vi "5_0_inverse FFT of one sided vs two sided spectrum.vi"() -> ()   [LabVIEW 2009]
uses:
  <vilib>/measure/matone.llb/Extract Single Tone Information 1 Chan.vi
  <vilib>/Analysis/2dsp.llb/Inverse Complex FFT.vi
  <vilib>/Analysis/2dsp.llb/Real FFT.vi
  <vilib>/Analysis/NI_AALBase.lvlib
  <vilib>/measure/NI_MAPro.lvlib
  <vilib>/Analysis/NI_AALPro.lvlib
panel:
  out "PHASE PLOT OF IFFT":dbl[](graph)=[-0.8524697408335709, -0.40748488207664046, -0.1268654978335297, 0.12686549783352957, 0.40748488207664024, 0.8524697408335707, 1.5889194659707906, 1.5966731628316637, 1.6041910783639635, 1.6118107017257388, 1.6197123575445933, 1.6280401156686646, 1.6369385301034163, 1.6465715078080854, 1.6571380811494125, 1.668890797356469, 1.6821610796097555, 1.6973972432967555, 1.715224596602943, 1.7365449259694004, 1.7627092545662675, 1.7958345210056603, 1.8394218293357656, 1.8996554825655303, 1.9883658653105416, 2.130300389496201, 2.380319581783001, 2.8348234385781517, 3.4483618686014315, 3.9028657253965804, 4.152884917683385, 4.294819441869041, 4.383529824614057, 4.443763477843824, 4.487350786173925, 4.520476052613318, 4.546640381210186, 4.567960710576643, 4.58578806388283, 4.60102422756983, 4.614294509823115, 4.626047226030174, 4.636613799371501, 4.64624677707617, 4.655145191510922, 4.6634729496349925, 4.671374605453847, 4.678994228815623, 4.6865121443479225, 4.694265841208795]
  out "PHASE PLOT OF IFFT":dbl[](graph)=[7.806255641895632e-18, -1.070222432237112e-16, -6.926012986585332e-17, -8.95286082736778e-17, -2.4757524506244172e-17, -7.708860338443508e-17, -1.1870100966642376e-16, -2.028583387333138e-17, -3.244626402670354e-17, -5.1237142864996e-17, -2.7729818653163923e-17, -3.052166662838311, -3.857180626159561, -3.4522573371371315, -2.9265484443936347, -3.332323038985992, -3.763563654552602, -6.34621297924532, -3.609239564041977, -1.9564428913976795, -1.3853313030041945, -3.745235757916132, -4.725507827503854, -5.486763286525393, -6.081674965765823, -6.218075312241696, -8.383184554491082, -6.174127459644382, -4.966447680000442, -6.573210745577857, -6.291926051943064, -6.7495541302012425, -6.759313157449682, -7.183594302336601, -6.596101120448532, -4.71238898038469, -6.242738848645043, -3.7248642537017105, -6.79886173291, -9.657554622227867, -7.853981633974483, -9.366981075199789, -9.552737084476966, -9.533582055953655, -9.277382354528344, -9.699789856635407, -7.853981633974483, -5.43623840730894, -7.060585609857342, -7.853981633974483, -6.7066247133393055, -6.738371234650006, -6.341312119269376, -6.200689197407941, -6.556801127375861, -7.853981633974483, -6.550303780412898, -6.35585762397127, -4.71238898038469, -3.6541253373308886, -4.71238898038469, -3.8318672767363133, -5.119942186117699, -3.710928254072696, -4.119135738411837, -3.7280195380119254, -4.2843202387005626, -1.9811033120489254, 0.689526342512747, -0.5330510016729039, 2.3244728172082056, 0.12183125310633174, -2.5660264286125947, -0.6175294809935509, -2.542876117116644, 0.0480981026284778, -1.3910453138610972, -3.2703822235332276, -2.884076452454559, -2.9596871114658927, -3.1595659301998222, -3.734802108132001, -3.5839862787232537, -3.8616075510042385, -3.6946513573707214, -4.71238898038469, -4.132634099636267, -6.053086329873605, -3.050702272396979, -3.737803844028845, -4.71238898038469, -5.601427829621794, -7.853981633974483, -6.530132536286139, -6.270083843304302, -6.450892009584458, -4.71238898038469, -2.7386471933636867, -2.0312901374214394, -3.9961826176864443]
  out "MAGNITUDE OF IFFT":dbl[](graph)=[0.01, 0.01, 0.01, 0.01, 0.01, 0.01, 0.01, 0.009999999999999998, 0.01, 0.01, 0.01, 1.1769286549004275e-18, 6.6460045320375995e-19, 1.3282359395858361e-18, 6.149476416360019e-19, 8.252020219132452e-19, 6.110656010294029e-19, 4.828187813833805e-19, 1.7839634152204216e-19, 1.266411875170956e-19, 3.615896476700937e-19, 3.9137843402403226e-19, 5.475363318400623e-19, 6.697102589357712e-19, 8.766988196791402e-19, 8.153536263231808e-19, 2.8656933719989682e-19, 6.348449873238717e-19, 5.516249800940764e-19, 4.568959162104949e-19, 1.0766538855279154e-18, 6.214814302944858e-19, 9.36869293875907e-19, 8.934827920481643e-19, 5.834435124906911e-19, 3.345487400322162e-20, 5.555658799234696e-19, 3.3253541146592564e-19, 3.1904450819839834e-19, 5.70498058306926e-19, 3.129593843111334e-19, 1.3900999350287225e-19, 2.798436470622704e-19, 9.77223791795179e-19, 9.820940712407218e-19, 4.3258949649040544e-19, 2.3589867581032264e-19, 2.0954758884453495e-19, 1.947105335811547e-19, 3.18890963982299e-19, 1.8998013584594692e-19, 1.2360817255724467e-18, 1.11210123854733e-18, 1.1140116385727674e-18, 1.1531188793745111e-18, 3.276667140500816e-19, 1.1510442472719137e-18, 1.1131611811269628e-18, 4.0650087380757416e-20, 1.2739142380935128e-18, 2.7729818653163923e-19, 1.2385093013585569e-18, 2.6191158553915634e-19, 6.569021055880242e-19, 6.516135414902478e-19, 7.161697525459617e-19, 7.517127896064829e-19, 2.8046798059658494e-19, 6.469331065721965e-19, 6.205367602260962e-19, 4.87382582781785e-19, 4.775392787866618e-19, 2.8336606694979876e-19, 1.440340997375154e-19, 8.810147345899317e-20, 3.0833776940221066e-19, 1.747274344599814e-19, 1.0334689731741024e-18, 1.6467217117304525e-19, 3.1673065223925814e-19, 5.236186963063961e-19, 6.6949404246627545e-19, 9.2136777446432e-19, 7.38380600284519e-19, 6.523649036422596e-19, 4.444643355793925e-19, 1.0133121096240545e-18, 1.4253454335586116e-18, 1.3935308412180152e-18, 6.708547467780006e-19, 3.129593843111334e-19, 8.936502141247432e-19, 3.1326666521253046e-19, 1.0018377239596355e-18, 4.16369368281998e-19, 7.037630734670443e-19, 2.3589867581032264e-19, 7.5430140173610385e-19, 3.122881064119443e-19, 4.227631070529326e-19]
  out "MAGNITUDE OF IFFT":dbl[](graph)=[0.030085439591800364, 0.021565797340465785, 0.01996041465777327, 0.019960414657773266, 0.02156579734046578, 0.030085439591800368, 0.011036219870674057, 0.007729782799349668, 0.005990078353216028, 0.004877706510838509, 0.00409027017264813, 0.0034957376876723805, 0.003025993855965793, 0.002641914167007991, 0.0023192569390351535, 0.0020421243943848154, 0.0017996178995784938, 0.0015839953294540714, 0.0013895964663497536, 0.0012121894116278009, 0.0010485639705040803, 0.0008962838542587668, 0.0007535610909382819, 0.000619264966236809, 0.0004931695725765839, 0.0003768139253352483, 0.0002762589760916794, 0.00020979442545002608, 0.00020979442545002614, 0.0002762589760916788, 0.0003768139253352492, 0.0004931695725765836, 0.00061926496623681, 0.0007535610909382812, 0.0008962838542587682, 0.0010485639705040805, 0.0012121894116277985, 0.001389596466349754, 0.0015839953294540714, 0.001799617899578496, 0.0020421243943848167, 0.002319256939035153, 0.0026419141670079908, 0.003025993855965793, 0.0034957376876723774, 0.004090270172648129, 0.0048777065108385085, 0.005990078353216027, 0.007729782799349666, 0.011036219870674059]
  out "IMAGINARY PART OF IFFT":dbl[](graph)=[-0.022651571147094166, -0.008546555734916897, -0.0025255006058700186, 0.002525500605870015, 0.008546555734916892, 0.022651571147094166, 0.011034407507150573, 0.0077271949713412814, 0.005986738567673323, 0.004873604498302707, 0.004085377593963007, 0.003490011745111045, 0.0030193772232602416, 0.002634333021058182, 0.0023106173956894526, 0.0020323070737813097, 0.001788469900357093, 0.0015713183012147198, 0.0013751284810124915, 0.001195576500966188, 0.0010293135577846436, 0.0008736845811875991, 0.0007265358337866712, 0.0005860794301187135, 0.00045079510569145584, 0.0003193567508704931, 0.00019057550176038718, 6.335377612981474e-05, -6.335377612981419e-05, -0.00019057550176038586, -0.00031935675087049384, -0.000450795105691455, -0.0005860794301187146, -0.0007265358337866712, -0.0008736845811876004, -0.0010293135577846436, -0.0011955765009661857, -0.001375128481012492, -0.0015713183012147196, -0.001788469900357095, -0.0020323070737813106, -0.002310617395689452, -0.0026343330210581817, -0.0030193772232602416, -0.0034900117451110418, -0.004085377593963006, -0.0048736044983027065, -0.0059867385676733225, -0.007727194971341279, -0.011034407507150573]
  out "IMAGINARY  PART OF IFFT":dbl[](graph)=[7.806255641895632e-20, -1.070222432237112e-18, -6.926012986585332e-19, -8.95286082736778e-19, -2.475752450624417e-19, -7.708860338443508e-19, -1.1870100966642376e-18, -2.0285833873331376e-19, -3.2446264026703544e-19, -5.1237142864996e-19, -2.7729818653163923e-19, -1.051077888933472e-19, 4.3601862232782005e-19, 4.0603052899077807e-19, -1.312240581677739e-19, 1.564385695482534e-19, 3.5603015337493493e-19, -3.0410800064616527e-20, 8.04187682809416e-20, -1.1734007814767696e-19, -3.5538860391659286e-19, 2.2216420822923857e-19, 5.474892158783854e-19, 4.787482065753655e-19, 1.7547068906596255e-19, 5.3050169237540845e-20, -2.4736944495925564e-19, 6.909766737395167e-20, 5.339179868407177e-19, -1.3066154122079454e-19, -9.410636981189501e-21, -2.7944655499562363e-19, -4.294057449873437e-19, -7.001162107709157e-19, -1.7960384507442347e-19, 3.345487400322162e-20, 2.2464546137888218e-20, 1.8314639527799346e-19, -1.5732832051499322e-19, 1.316025965929817e-19, -3.129593843111334e-19, -8.029872339970768e-21, 3.5710909056241305e-20, 1.0611628763201875e-19, -1.4423277025846226e-19, 1.1747330538880442e-19, -2.3589867581032264e-19, 1.5700602710305712e-19, -1.365755924152834e-19, -3.18890963982299e-19, -7.806255641895632e-20, -5.434177655232912e-19, -6.460650408956147e-20, 9.179742081208677e-20, -3.115894503382571e-19, -3.276667140500816e-19, -3.038218141772169e-19, -8.082481524967397e-20, 4.0650087380757416e-20, 6.247097899101185e-19, 2.7729818653163923e-19, 7.886195098672507e-19, 2.404592958546189e-19, 3.5411790700049025e-19, 5.402699299637449e-19, 3.9632005538727372e-19, 6.838850975765389e-19, -2.5718869294115346e-19, 4.115606017225533e-19, -3.1533407612639655e-19, 3.5538860391659286e-19, 5.803539126420531e-20, -1.542389485149524e-19, -8.339901148187951e-20, -4.9652468088997603e-20, 1.482474413875035e-20, -1.7191226768039992e-19, 1.3273238009293602e-19, -4.1938616837222844e-20, -5.729784281695019e-20, 9.410636981189501e-21, 3.742639199761009e-19, 3.944411183458555e-19, 4.868851196889971e-19, 3.4268232578033095e-19, 4.444643355793925e-19, 8.477338263917479e-19, 3.250840823220212e-19, -1.264842323712848e-19, 3.766925804586781e-19, 3.129593843111334e-19, 5.631413846525491e-19, -3.1326666521253046e-19, -2.448941657101633e-19, 5.4548921803176945e-21, -1.1747330538880442e-19, 2.3589867581032264e-19, -2.9578390518120167e-19, -2.7975804181915034e-19, 3.18890963982299e-19]
  out "REAL PART OF IFFT":dbl[](graph)=[0.0198, 0.019800000000000005, 0.019800000000000005, 0.0198, 0.019800000000000005, 0.019800000000000005, -0.0001999999999999994, -0.0002000000000000014, -0.00019999999999999952, -0.00019999999999999977, -0.00020000000000000063, -0.00020000000000000196, -0.00020000000000000142, -0.000200000000000001, -0.0002000000000000014, -0.00019999999999999844, -0.00019999999999999952, -0.00019999999999999855, -0.00019999999999999955, -0.00020000000000000123, -0.00020000000000000234, -0.00019999999999999952, -0.00020000000000000004, -0.00020000000000000047, -0.00019999999999999898, -0.00019999999999999968, -0.00019999999999999944, -0.00019999999999999966, -0.0001999999999999999, -0.00019999999999999985, -0.00020000000000000025, -0.00020000000000000017, -0.00020000000000000017, -0.00019999999999999795, -0.00020000000000000017, -0.0002000000000000035, -0.00020000000000000052, -0.0001999999999999996, -0.0002000000000000001, -0.0001999999999999999, -0.00020000000000000196, -0.00020000000000000074, -0.00020000000000000074, -0.00020000000000000074, -0.00020000000000000074, -0.00020000000000000185, -0.000200000000000002, -0.00020000000000000172, -0.00020000000000000177, -0.00020000000000000302]
  out "REAL PART OF IFFT":dbl[](graph)=[0.01, 0.01, 0.01, 0.01, 0.01, 0.01, 0.01, 0.009999999999999998, 0.01, 0.01, 0.01, -1.1722258363641714e-18, -5.015790300461065e-19, -1.2646540715685605e-18, -6.007835288285301e-19, -8.102378360255736e-19, -4.966323576341414e-19, 4.818601030340264e-19, -1.5924219408380846e-19, -4.763713295358185e-20, 6.667843360785852e-20, -3.222113331355359e-19, 7.182839392716467e-21, 4.683075758779576e-19, 8.589591711516409e-19, 8.136259678145908e-19, -1.446732273910345e-19, 6.310734270223439e-19, 1.3864235280658389e-19, 4.378143897768028e-19, 1.0766127572781059e-18, 5.551115123125783e-19, 8.326672684688674e-19, 5.551115123125783e-19, 5.551115123125783e-19, 0.0, 5.551115123125783e-19, -2.7755575615628914e-19, 2.7755575615628914e-19, -5.551115123125783e-19, 0.0, -1.3877787807814457e-19, -2.7755575615628914e-19, -9.71445146547012e-19, -9.71445146547012e-19, -4.163336342344337e-19, 0.0, 1.3877787807814457e-19, 1.3877787807814457e-19, 0.0, 1.7320129705455935e-19, 1.1102230246251566e-18, 1.1102230246251566e-18, 1.1102230246251566e-18, 1.1102230246251566e-18, 0.0, 1.1102230246251566e-18, 1.1102230246251566e-18, 0.0, -1.1102230246251566e-18, 0.0, -9.549788260523884e-19, 1.0381235801548705e-19, -5.53281921146509e-19, -3.642919299551295e-19, -5.965144827743685e-19, -3.1204693776848427e-19, -1.11876111673348e-19, 4.991395751580141e-19, 5.344439083995734e-19, -3.335276933108533e-19, 4.739996372835065e-19, -2.3771132631744684e-19, 1.174326478073362e-19, -7.277707082808949e-20, 3.079811796216636e-19, 3.12385750947386e-20, -1.0249098661777034e-18, -1.5924219408380846e-19, -3.115048366822415e-19, -5.23534124038938e-19, -5.551115123125783e-19, -8.326672684688674e-19, -5.551115123125783e-19, -5.551115123125783e-19, 0.0, -5.551115123125783e-19, 1.3877787807814458e-18, -1.3877787807814458e-18, -5.551115123125783e-19, 0.0, 6.938893903907229e-19, 0.0, 9.71445146547012e-19, 4.163336342344337e-19, 6.938893903907229e-19, 0.0, -6.938893903907229e-19, -1.3877787807814457e-19, -2.7755575615628914e-19]
  out "FREQ":dbl=0.049366588097272006 format="%.2p"
  out "FREQ":dbl=0.02469635114895025 format="%.2p"
  out "?":bool
  out "?":bool
  out "INVERSE FFT OF ONE SIDED SPECTRUM":cluster{i32, dbl, dbl[]}(graph)={0, 0.001, [0.0198, 0.019800000000000005, 0.019800000000000005, 0.0198, 0.019800000000000005, 0.019800000000000005, -0.0001999999999999994, -0.0002000000000000014, -0.00019999999999999952, -0.00019999999999999977, -0.00020000000000000063, -0.00020000000000000196, -0.00020000000000000142, -0.000200000000000001, -0.0002000000000000014, -0.00019999999999999844, -0.00019999999999999952, -0.00019999999999999855, -0.00019999999999999955, -0.00020000000000000123, -0.00020000000000000234, -0.00019999999999999952, -0.00020000000000000004, -0.00020000000000000047, -0.00019999999999999898, -0.00019999999999999968, -0.00019999999999999944, -0.00019999999999999966, -0.0001999999999999999, -0.00019999999999999985, -0.00020000000000000025, -0.00020000000000000017, -0.00020000000000000017, -0.00019999999999999795, -0.00020000000000000017, -0.0002000000000000035, -0.00020000000000000052, -0.0001999999999999996, -0.0002000000000000001, -0.0001999999999999999, -0.00020000000000000196, -0.00020000000000000074, -0.00020000000000000074, -0.00020000000000000074, -0.00020000000000000074, -0.00020000000000000185, -0.000200000000000002, -0.00020000000000000172, -0.00020000000000000177, -0.00020000000000000302]}
  out "INVERSE FFT OF TWO SIDED SPECTRUM":cluster{"index":i32, dbl, dbl[]}(graph)={"index"=0, 0.001, [0.01, 0.01, 0.01, 0.01, 0.01, 0.01, 0.01, 0.009999999999999998, 0.01, 0.01, 0.01, -1.1722258363641714e-18, -5.015790300461065e-19, -1.2646540715685605e-18, -6.007835288285301e-19, -8.102378360255736e-19, -4.966323576341414e-19, 4.818601030340264e-19, -1.5924219408380846e-19, -4.763713295358185e-20, 6.667843360785852e-20, -3.222113331355359e-19, 7.182839392716467e-21, 4.683075758779576e-19, 8.589591711516409e-19, 8.136259678145908e-19, -1.446732273910345e-19, 6.310734270223439e-19, 1.3864235280658389e-19, 4.378143897768028e-19, 1.0766127572781059e-18, 5.551115123125783e-19, 8.326672684688674e-19, 5.551115123125783e-19, 5.551115123125783e-19, 0.0, 5.551115123125783e-19, -2.7755575615628914e-19, 2.7755575615628914e-19, -5.551115123125783e-19, 0.0, -1.3877787807814457e-19, -2.7755575615628914e-19, -9.71445146547012e-19, -9.71445146547012e-19, -4.163336342344337e-19, 0.0, 1.3877787807814457e-19, 1.3877787807814457e-19, 0.0, 1.7320129705455935e-19, 1.1102230246251566e-18, 1.1102230246251566e-18, 1.1102230246251566e-18, 1.1102230246251566e-18, 0.0, 1.1102230246251566e-18, 1.1102230246251566e-18, 0.0, -1.1102230246251566e-18, 0.0, -9.549788260523884e-19, 1.0381235801548705e-19, -5.53281921146509e-19, -3.642919299551295e-19, -5.965144827743685e-19, -3.1204693776848427e-19, -1.11876111673348e-19, 4.991395751580141e-19, 5.344439083995734e-19, -3.335276933108533e-19, 4.739996372835065e-19, -2.3771132631744684e-19, 1.174326478073362e-19, -7.277707082808949e-20, 3.079811796216636e-19, 3.12385750947386e-20, -1.0249098661777034e-18, -1.5924219408380846e-19, -3.115048366822415e-19, -5.23534124038938e-19, -5.551115123125783e-19, -8.326672684688674e-19, -5.551115123125783e-19, -5.551115123125783e-19, 0.0, -5.551115123125783e-19, 1.3877787807814458e-18, -1.3877787807814458e-18, -5.551115123125783e-19, 0.0, 6.938893903907229e-19, 0.0, 9.71445146547012e-19, 4.163336342344337e-19, 6.938893903907229e-19, 0.0, -6.938893903907229e-19, -1.3877787807814457e-19, -2.7755575615628914e-19]}
  out "?":string="SAMPLE"
  in  "stop":bool
  out "DETECTED FREQUENCY":dbl=0.024696351148950267 format="%.2p"
  out "ONE SIDED FFT MAG PLOT":cluster{i32, dbl, dbl[]}(graph)={0, 10.0, [0.11, 0.2156827343158089, 0.20303192091000685, 0.1829258216733136, 0.156748090317914, 0.12627503029350087, 0.09353191720116408, 0.06063097450005466, 0.029605108344486146, 0.002251739098357606, 0.02, 0.03618768475694426, 0.045871861539495615, 0.04914626439933461, 0.04660229940576391, 0.03925221011010302, 0.028418967730971842, 0.015603755543126093, 0.0023436871809210187, 0.009927036344868552, 0.02, 0.026988776498658107, 0.03039054622059342, 0.03010869808349327, 0.026435786365307575, 0.02, 0.011681690419824685, 0.002509183429725328, 0.006455174897940613, 0.014227167303847467, 0.02, 0.023221284976236406, 0.023640737165832135, 0.02132473138039944, 0.016637294774129143, 0.01019050898988858, 0.002770324632154191, 0.004753846731831293, 0.011525926996682445, 0.016796071052742112, 0.02, 0.02081668504695303, 0.019198691928627776, 0.015372439512982547, 0.00980881455489394, 0.003167688806490725, 0.003777412316085198, 0.01022621260854057, 0.015440733616207286, 0.01882690532036019]}
  out "# OF CYCLES":dbl=5.0
  in  "?":bool
  out "TWO SIDED FFT MAG PLOT":cluster{"index":i32, dbl, dbl[]}(graph)={"index"=0, 10.0, [0.11, 0.10784136715790445, 0.10151596045500343, 0.0914629108366568, 0.078374045158957, 0.06313751514675044, 0.04676595860058204, 0.03031548725002733, 0.014802554172243073, 0.001125869549178803, 0.01, 0.01809384237847213, 0.022935930769747807, 0.024573132199667305, 0.023301149702881954, 0.01962610505505151, 0.014209483865485921, 0.0078018777715630466, 0.0011718435904605094, 0.004963518172434276, 0.01, 0.013494388249329053, 0.01519527311029671, 0.015054349041746636, 0.013217893182653788, 0.01, 0.005840845209912343, 0.001254591714862664, 0.0032275874489703063, 0.0071135836519237335, 0.01, 0.011610642488118203, 0.011820368582916067, 0.01066236569019972, 0.008318647387064572, 0.00509525449494429, 0.0013851623160770956, 0.0023769233659156467, 0.005762963498341223, 0.008398035526371056, 0.01, 0.010408342523476515, 0.009599345964313888, 0.0076862197564912735, 0.00490440727744697, 0.0015838444032453625, 0.001888706158042599, 0.005113106304270285, 0.007720366808103643, 0.009413452660180096, 0.01, 0.009413452660180096, 0.007720366808103643, 0.005113106304270285, 0.001888706158042599, 0.0015838444032453625, 0.00490440727744697, 0.0076862197564912735, 0.009599345964313888, 0.010408342523476515, 0.01, 0.008398035526371056, 0.005762963498341223, 0.0023769233659156467, 0.0013851623160770956, 0.00509525449494429, 0.008318647387064572, 0.01066236569019972, 0.011820368582916067, 0.011610642488118203, 0.01, 0.0071135836519237335, 0.0032275874489703063, 0.001254591714862664, 0.005840845209912343, 0.01, 0.013217893182653788, 0.015054349041746636, 0.01519527311029671, 0.013494388249329053, 0.01, 0.004963518172434276, 0.0011718435904605094, 0.0078018777715630466, 0.014209483865485921, 0.01962610505505151, 0.023301149702881954, 0.024573132199667305, 0.022935930769747807, 0.01809384237847213, 0.01, 0.001125869549178803, 0.014802554172243073, 0.03031548725002733, 0.04676595860058204, 0.06313751514675044, 0.078374045158957, 0.0914629108366568, 0.10151596045500343, 0.10784136715790445]}
  in  "Delta t":dbl=0.1 format="%0.2f"
  in  "Duty cycle (%)":dbl=50.0 format="%0.2f"
  in  "Width":i32=11
  in  "Start":dbl format="%0.2f"
  in  "End":dbl=1.0 format="%0.2f"
  out "TIME DOMAIN ORIGINAL SIGNAL":T1(graph)={0, "# OF SAMPLES"=1.0, "Sinc Pattern"=[1.0, 1.0, 1.0, 1.0, 1.0, 1.0, 1.0, 1.0, 1.0, 1.0, 1.0, 0.0, 0.0, 0.0, 0.0, 0.0, 0.0, 0.0, 0.0, 0.0, 0.0, 0.0, 0.0, 0.0, 0.0, 0.0, 0.0, 0.0, 0.0, 0.0, 0.0, 0.0, 0.0, 0.0, 0.0, 0.0, 0.0, 0.0, 0.0, 0.0, 0.0, 0.0, 0.0, 0.0, 0.0, 0.0, 0.0, 0.0, 0.0, 0.0, 0.0, 0.0, 0.0, 0.0, 0.0, 0.0, 0.0, 0.0, 0.0, 0.0, 0.0, 0.0, 0.0, 0.0, 0.0, 0.0, 0.0, 0.0, 0.0, 0.0, 0.0, 0.0, 0.0, 0.0, 0.0, 0.0, 0.0, 0.0, 0.0, 0.0, 0.0, 0.0, 0.0, 0.0, 0.0, 0.0, 0.0, 0.0, 0.0, 0.0, 0.0, 0.0, 0.0, 0.0, 0.0, 0.0, 0.0, 0.0, 0.0, 0.0]}
  in  "Reset phase":bool=TRUE
  in  "DELAY":dbl(knob) min=0.0 max=10.0 scale=0.0..10.0
  in  "SAMPLING\nFREQUENCY (Hz)":dbl(slide)=1000.0 scale=0.0..20000.0 scale format="%#_6p"
  in  "# OF SAMPLES":dbl=100.0
  in  "AMPLITUDE":dbl=1.0
  in  "PHASE IN":dbl(knob) scale=0.0..180.0
  in  "SIGNAL FREQUENCY":dbl(knob)=50.0 scale=0.0..10000.0 scale format="%#_6p"
  in  "SIGNAL":T2(ring)=enum."PULSE"
  # "SAMPLING INFO"
  # "ORIGINAL SIGNAL \nCHARACTERISTICS"
  # "RAMP"
  # "PULSE"
  # "SQUARE"
  # "SINC"
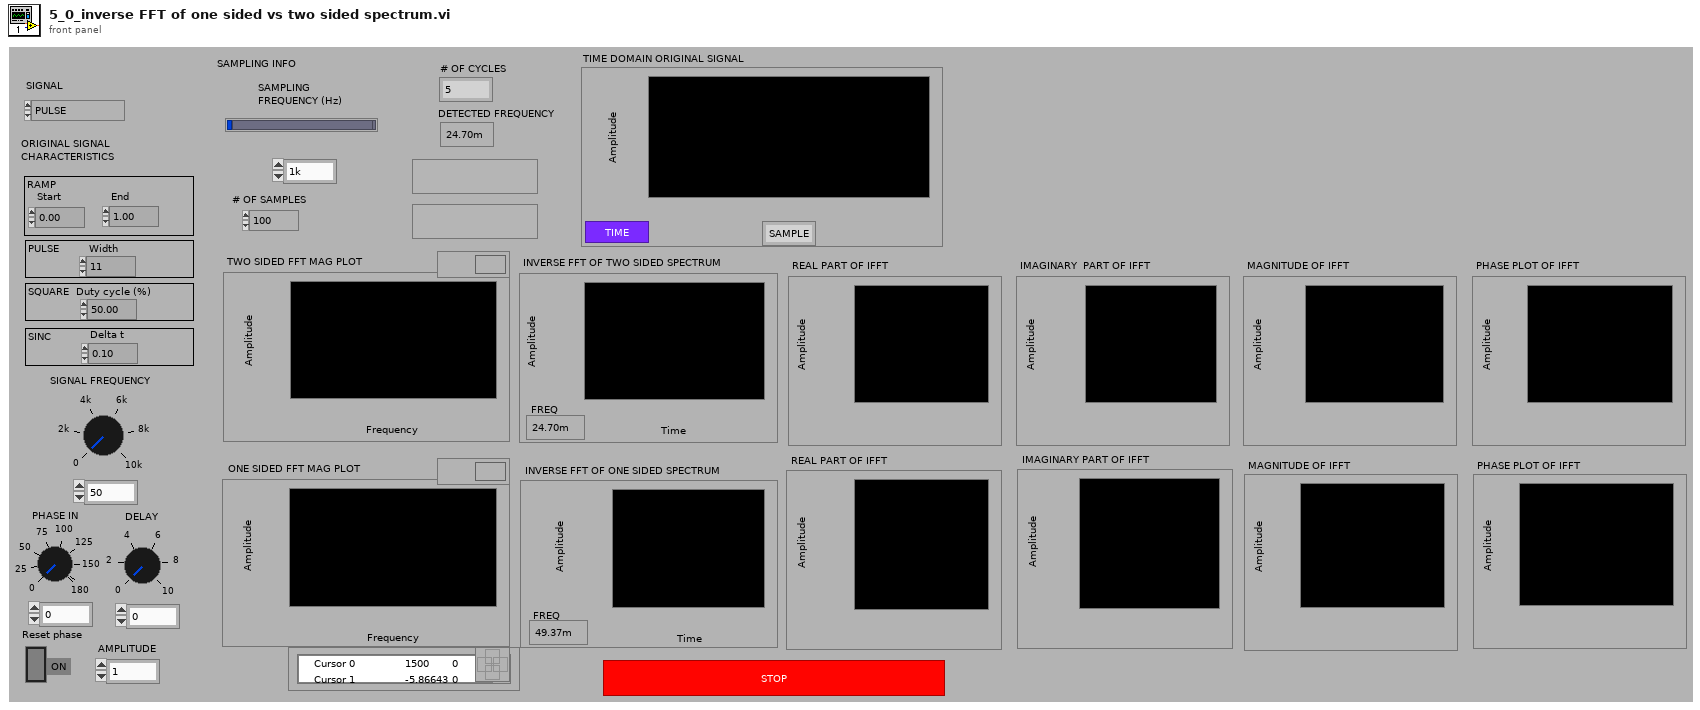
[diagram p1: front panel]
types:
  T1 = cluster{i32, "# OF SAMPLES":dbl, "Sinc Pattern":dbl[]}
  T2 = enum16{"SINE", "TRIANGULAR", "RAMP", "IMPULSE", "SINC ", "PULSE", "SQUARE"}
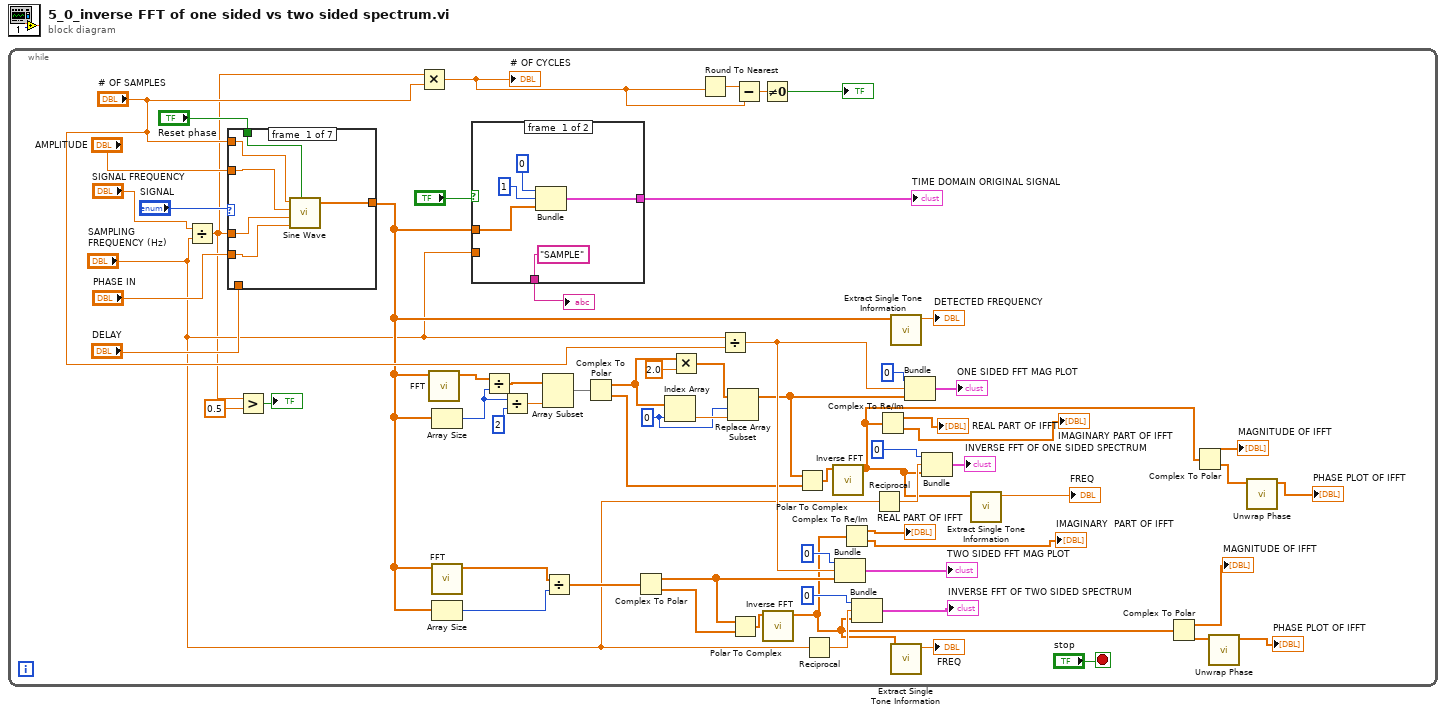
[diagram p0: block diagram]
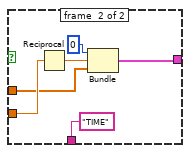
[diagram p2: hidden frame]
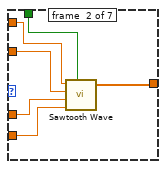
[diagram p3: hidden frame]
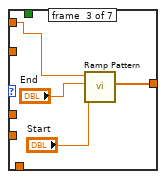
[diagram p4: hidden frame]
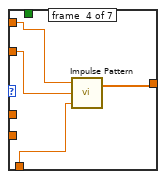
[diagram p5: hidden frame]
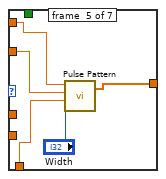
[diagram p6: hidden frame]
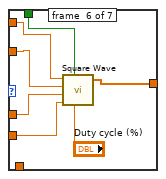
[diagram p7: hidden frame]
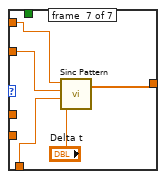
[diagram p8: hidden frame]
diagram:
  n1 = while {
    stop <- "stop" stop-if-true
    w52 = 0 ("index")
    n2 = Divide(x="SIGNAL FREQUENCY", y="SAMPLING\nFREQUENCY (Hz)") -> (x/y=w20:dbl)
    n3 = case shown="\"RAMP\"" "SIGNAL" {
      tunnel: "Reset phase" -> [w83 w89 _ _ _ w109 _]
      tunnel: "AMPLITUDE" -> [w81 w87 _ w96 w101 w107 w113]
      tunnel: "# OF SAMPLES" -> [w82 w88 w92 w97 w102 w108 w114]
      tunnel: w20 -> [w80 w86 _ _ _ w106 _]
      tunnel: "PHASE IN" -> [w79 w85 _ _ _ w105 _]
      tunnel: "DELAY" -> [_ _ _ w95 w100 _ w112]
      tunnel: [w78 w84 w93 w94 w99 w104 w111] -> w38
      frame #0 {
        n4 = call <vilib>:"Sine Wave.vi"("samples"=w82, "amplitude"=w81, "frequency"=w80, "phase in"=w79, "reset phase"=w83) -> ("sine wave"=w78:dbl[])  [unwired: 2 out]
      }
      frame #1 {
        n5 = call <vilib>:"Sawtooth Wave.vi"("samples"=w88, "amplitude"=w87, "frequency"=w86, "phase in"=w85, "reset phase"=w89) -> ("sawtooth wave"=w84:dbl[])  [unwired: 2 out]
      }
      frame #2 {
        n6 = call <vilib>:"Ramp Pattern.vi"("start"="Start", "end"="End", "samples"=w92) -> ("Ramp Pattern"=w93:dbl[])  [unwired: 7 in, 1 out]
      }
      frame #3 {
        n7 = call <vilib>:"Impulse Pattern.vi"("delay"=w95, "amplitude"=w96, "samples"=w97) -> ("Impulse Pattern"=w94:dbl[])  [unwired: 1 out]
      }
      frame #4 {
        n8 = call <vilib>:"Pulse Pattern.vi"("width"="Width", "delay"=w100, "amplitude"=w101, "samples"=w102) -> ("Pulse Pattern"=w99:dbl[])  [unwired: 1 out]
      }
      frame #5 {
        n9 = call <vilib>:"Square Wave.vi"("samples"=w108, "reset phase"=w109, "amplitude"=w107, "frequency"=w106, "duty cycle (%)"="Duty cycle (%)", "phase in"=w105) -> ("square wave"=w104:dbl[])  [unwired: 2 out]
      }
      frame #6 {
        n10 = call <vilib>:"Sinc Pattern.vi"("delta t"="Delta t", "delay"=w112, "amplitude"=w113, "samples"=w114) -> ("Sinc Pattern"=w111:dbl[])  [unwired: 1 out]
      }
    }
    n11 = Greater?(x=w20, y=0.5) -> (0:→"?":bool)
    n12 = Multiply(x=w20, y="# OF SAMPLES") -> (x*y=w17:dbl)
    "# OF CYCLES" <- w17
    n13 = call-poly <vilib>:"FFT.vi"("X"=w38) -> ("FFT {X}"=w58:cdb[])  [unwired: 9 in, 1 out]
    n14 = Array Size(array=w38) -> (size(s)=w56:i32)
    n15 = call-poly <vilib>:"FFT.vi"("X"=w38) -> ("FFT {X}"=w36:cdb[])  [unwired: 9 in, 1 out]
    n16 = Array Size(array=w38) -> (size(s)=w35:i32)
    n17 = case shown="True" "?" {
      tunnel: w38 -> [w70 w75]
      tunnel: [w68 w73] -> w59
      tunnel: "SAMPLING\nFREQUENCY (Hz)" -> [_ w77]
      tunnel: ["SAMPLE" "TIME"] -> w45
      frame #0 {
        n18 = Bundle(0, 1, "Sinc Pattern"=w70) -> (w68:cluster{i32, i32, "Sinc Pattern":dbl[]})  [unwired: 1 in]
      }
      frame #1 {
        n19 = Reciprocal(x=w77) -> (1/x=w76:dbl)
        n20 = Bundle(0, w76, "Sinc Pattern"=w75) -> (w73:cluster{i32, dbl, "Sinc Pattern":dbl[]})  [unwired: 1 in]
      }
    }
    "TIME DOMAIN ORIGINAL SIGNAL" <- w59
    "?" <- w45
    n21 = Divide(x=w58, y=w56) -> (x/y=w40:cdb[])
    n22 = Divide(x=w56, y=2) -> (x/y=w57:dbl)
    n23 = Array Subset(array=w40, length=w57) -> (w54:cdb[])  [unwired: 1 in]
    n24 = Divide(x=w36, y=w35) -> (x/y=w37:cdb[])
    n25 = Complex To Polar(r * e^(i*theta)=w54) -> (r=w43:dbl[], theta=w22:dbl[])
    n26 = Complex To Polar(r * e^(i*theta)=w37) -> (r=w34:dbl[], theta=w33:dbl[])
    n27 = Index Array(array=w43, index=w52) -> (element=w53:dbl)
    n28 = Multiply(x=w43, y=2.0) -> (x*y=w51:dbl[])
    n29 = Round To Nearest(number=w17) -> (nearest integer value=w18:dbl)
    n30 = Divide(x="SAMPLING\nFREQUENCY (Hz)", y="# OF SAMPLES") -> (x/y=w41:dbl)
    n31 = Replace Array Subset(array=w51, new element=w53, index=w52) -> (w26:dbl[])
    n32 = Polar To Complex(1:w33, 2:w34) -> (0:w32:cdb[])
    n33 = Subtract(x=w18, y=w17) -> (x-y=w16:dbl)
    n34 = Not Equal To 0?(x=w16) -> (x != 0?=→"?":bool)
    n35 = call-poly <vilib>:"Inverse FFT.vi"("FFT {X}"=w32) -> ("X"=w6:cdb[])  [unwired: 9 in, 1 out]
    n36 = Polar To Complex(1:w22, 2:w26) -> (0:w25:cdb[])
    n37 = Reciprocal(x="SAMPLING\nFREQUENCY (Hz)") -> (1/x=w30:dbl)
    n38 = call-poly <vilib>:"Inverse FFT.vi"("FFT {X}"=w25) -> ("X"=w8:cdb[])  [unwired: 9 in, 1 out]
    n39 = Bundle("index"=0, w41, w34) -> (→"TWO SIDED FFT MAG PLOT":cluster{"index":i32, dbl, dbl[]})  [unwired: 1 in]
    n40 = Complex To Re/Im(x + iy=w6) -> (x=→"REAL PART OF IFFT":dbl[], y=→"IMAGINARY  PART OF IFFT":dbl[])
    n41 = Bundle("index"=0, w30, "X"=w6) -> (→"INVERSE FFT OF TWO SIDED SPECTRUM":cluster{"index":i32, dbl, "X":cdb[]})  [unwired: 1 in]
    n42 = Reciprocal(x="SAMPLING\nFREQUENCY (Hz)") -> (1/x=w28:dbl)
    n43 = Complex To Re/Im(x + iy=w8) -> (x=→"REAL PART OF IFFT":dbl[], y=→"IMAGINARY PART OF IFFT":dbl[])
    n44 = call-poly <vilib>:"Extract Single Tone Information.vi"("time signal in"=w38) -> ("detected frequency"=→"DETECTED FREQUENCY":dbl)  [unwired: 5 in, 5 out]
    n45 = call-poly <vilib>:"Extract Single Tone Information.vi"("time signal in"=w6) -> ("detected frequency"=→"FREQ":dbl)  [unwired: 5 in, 5 out]
    n46 = Bundle(0, w41, w26) -> (→"ONE SIDED FFT MAG PLOT":cluster{i32, dbl, dbl[]})  [unwired: 1 in]
    n47 = Bundle("index"=0, w28, "X"=w8) -> (→"INVERSE FFT OF ONE SIDED SPECTRUM":cluster{"index":i32, dbl, "X":cdb[]})  [unwired: 1 in]
    n48 = call-poly <vilib>:"Extract Single Tone Information.vi"("time signal in"=w8) -> ("detected frequency"=→"FREQ":dbl)  [unwired: 5 in, 5 out]
    n49 = Complex To Polar(r * e^(i*theta)=w6) -> (r=→"MAGNITUDE OF IFFT":dbl[], theta=w4:dbl[])
    n50 = Complex To Polar(r * e^(i*theta)=w8) -> (r=→"MAGNITUDE OF IFFT":dbl[], theta=w2:dbl[])
    n51 = call <vilib>:"Unwrap Phase.vi"("Phase"=w4) -> ("Unwrapped Phase"=→"PHASE PLOT OF IFFT":dbl[])  [unwired: 9 in, 1 out]
    n52 = call <vilib>:"Unwrap Phase.vi"("Phase"=w2) -> ("Unwrapped Phase"=→"PHASE PLOT OF IFFT":dbl[])  [unwired: 9 in, 1 out]
  }
